vi "test_data item filter.vi"(7 "data items":string[](array[string]), 8 "error in":errorcluster, 9 "match behavior":T4, 10 "aggregation method":T5=enum."All", 11 "directory":path) -> (0 "error out":errorcluster, 3 "failure info":T1 {"Log Record"."timestamp" format="%<%x %.3X>T"})   [LabVIEW 2018]
uses:
  api/extension/filter_interface/Aggregation Method.ctl
  api/extension/filter_interface/Match Behavior.ctl
  api/Failure Information.ctl
  api/Log Record.ctl
  api/logger_class/Internal Log Levels.ctl
  api/Log Levels.ctl
  api/configuration/formatters/format_string_formatter/Format String.lvclass
  C:/Users/Colin/Documents/software_projects/labview/glog/src/api/extension/formatter_interface/Formatter.lvclass
  api/configuration/filters/data_item_filter/Data Item.lvclass
  C:/Users/Colin/Documents/software_projects/labview/glog/src/api/extension/filter_interface/Filter.lvclass
  api/configuration/handlers/file_handler/File Handler.lvclass
  C:/Users/Colin/Documents/software_projects/labview/glog/src/api/extension/formatting_handler_interface/Formatting Handler.lvclass
  api/configuration/filters/data_item_filter/New (Array).vi
  api/logger_class/Log (Parts).vi
  api/logger_class/Logger.lvclass
  api/GLog.lvlib
panel:
  # "Connector Pane"
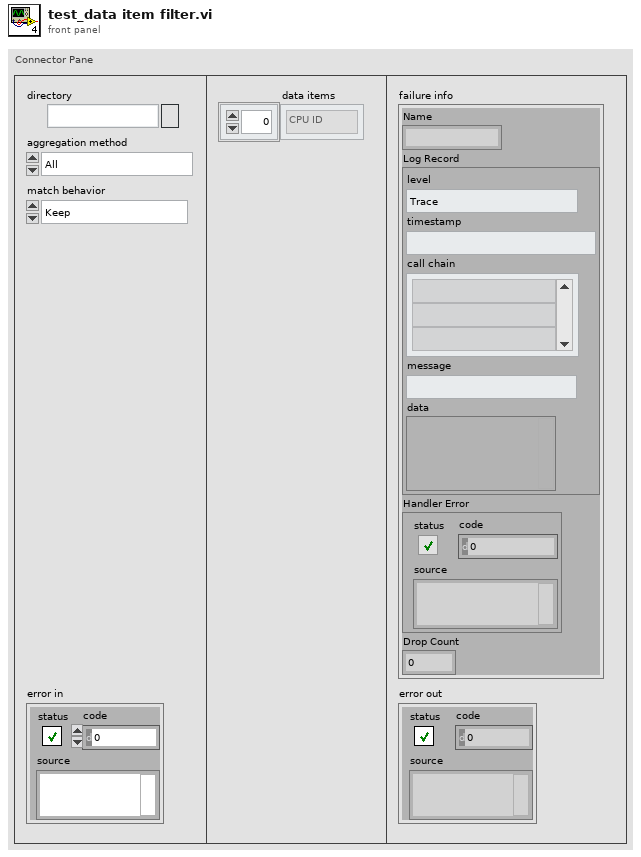
[diagram p1: front panel]
types:
  T1 = typedef "GLog.lvlib/Failure Information.ctl" = cluster{"Name":string, "Log Record":T2, "Handler Error":errorcluster, "Drop Count":u32}
  T2 = typedef "GLog.lvlib/Log Record.ctl" = cluster{"level":T3, "timestamp":timestamp, "call chain":string[], "message":string, "data":variant}
  T3 = typedef "GLog.lvlib/Internal Log Levels.ctl" = enum16{"Trace", "Debug", "Info", "Warning", "Error", "Critical", "Internal"}
  T4 = typedef "GLog.lvlib/Match Behavior.ctl" = enum16{"Keep", "Discard"}
  T5 = typedef "GLog.lvlib/Aggregation Method.ctl" = enum16{"Any", "Only", "All", "None"}
  T6 = typedef "GLog.lvlib/Log Levels.ctl" = enum16{"Trace", "Debug", "Info", "Warning", "Error", "Critical"}
  T7 = cluster{"Iteration":i32, "CPU ID":string, "Machine Name":string, "PID":string}
  T8 = cluster{"Iteration":i32, "CPU ID":string, "Machine Name":string}
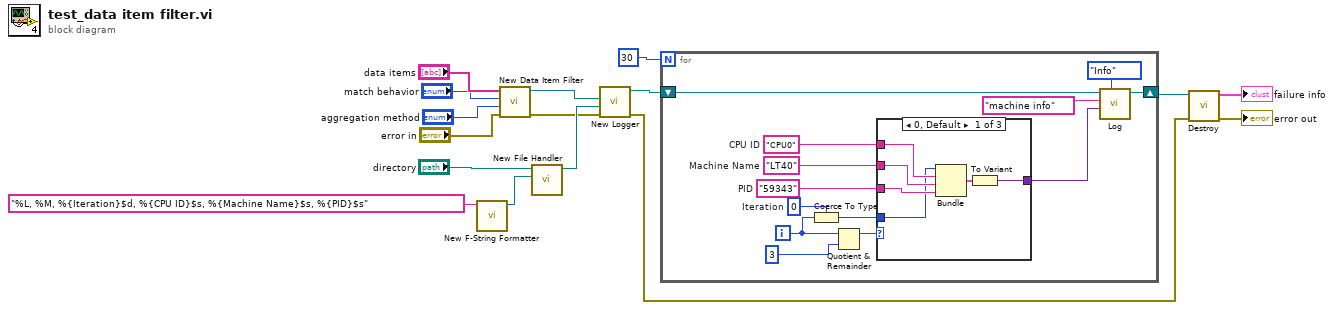
[diagram p0: block diagram]
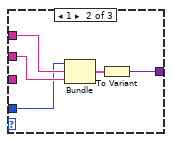
[diagram p2: hidden frame]
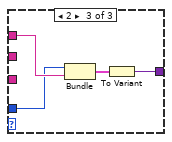
[diagram p3: hidden frame]
diagram:
  n1 = call "New F-String Formatter.vi"("format string (\"%T | %L | %M\")"="%L, %M, %{Iteration}$d, %{CPU ID}$s, %{Machine Name}$s, %{PID}$s" ("format string (\"%T | %L | %M\")")) -> ("new f-string formatter"=w8:refnum<class "Format String.lvclass">)  [unwired: 10 in]
  n2 = call-poly "New Data Item Filter.vi"("error in (no error)"="error in", "aggregation method (all)"="aggregation method", "match behavior (keep)"="match behavior", "data item names"="data items") -> ("error out"=w12:errorcluster, "data item out"=w1:refnum<class "Data Item.lvclass">)  [unwired: 6 in]
  n3 = call "New File Handler.vi"("formatter (JSON)"=w8, "log directory (<app dir>/logs)"="directory") -> ("file handler"=w14:refnum<class "File Handler.lvclass">)  [unwired: 9 in]
  n4 = call "New Logger.vi"("error in (no error)"=w12, "log handler (file handler)"=w14, "log filter (none)"=w1) -> ("error out"=w4:errorcluster, "logger"=w9:refnum<class "Logger.lvclass">)  [unwired: 7 in]
  n5 = for {
    N: 30 -> [_]
    shift-right: [w28] -> w5
    shift-left: w9 -> [w29]
    i -> [w20]
    w22 = 0  # Iteration
    w23 = "59343"  # PID
    w24 = "LT40"  # Machine Name
    w25 = "CPU0"  # CPU ID
    n6 = Coerce To Type(0:w20, 1:w22) -> (2:w21:i32)
    n7 = Quotient & Remainder(x=w20, y=3) -> (x-y*floor(x/y)=w26:i32)  [unwired: 1 out]
    n8 = case shown="0, Default" w26 {
      tunnel: w25 -> [w35 w39 w43]
      tunnel: w24 -> [w34 w38 _]
      tunnel: w23 -> [w33 _ _]
      tunnel: [w31 w37 w42] -> w18
      tunnel: w21 -> [w30 w36 w41]
      frame 0, Default {
        n9 = Bundle("Iteration"=w30, "CPU ID"=w35, "Machine Name"=w34, "PID"=w33) -> (w32:T7)  [unwired: 1 in]
        n10 = To Variant(anything=w32) -> (Variant=w31:variant)
      }
      frame 1 {
        n11 = Bundle("Iteration"=w36, "CPU ID"=w39, "Machine Name"=w38) -> (w40:T8)  [unwired: 1 in]
        n12 = To Variant(anything=w40) -> (Variant=w37:variant)
      }
      frame 2 {
        n13 = Bundle("Iteration"=w41, "CPU ID"=w43) -> (w44:cluster{"Iteration":i32, "CPU ID":string})  [unwired: 1 in]
        n14 = To Variant(anything=w44) -> (Variant=w42:variant)
      }
    }
    n15 = call-poly "Log.vi"("log level"=Log_Levels."Info", "data (null)"=w18, "message"="machine info", "logger in"=w29) -> ("logger out"=w28:refnum<class "Logger.lvclass">)  [unwired: 7 in]
  }
  n16 = call "Destroy.vi"("error in (no error)"=w4, "logger in"=w5) -> ("error out"=→"error out":errorcluster, "failure info"=→"failure info":T1)  [unwired: 8 in]
